vi "Pressure Generator.vi"() -> (2 "Trend Parameters":T1)   [LabVIEW 2015]
uses:
  Controls/Trend Parameters.ctl
panel:
  out "Frequency (Hz)":dbl[](array[numeric])
  out "DC":dbl[](array[numeric])
  out "Amplitude":dbl[](array[numeric])
  out "Noise Level":dbl[](array[numeric])
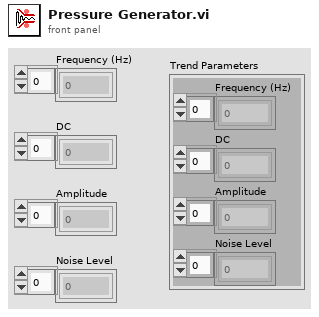
[diagram p1: front panel]
types:
  T1 = typedef "Trend Parameters.ctl" = cluster{"Frequency (Hz)":dbl[], "DC":dbl[], "Amplitude":dbl[], "Noise Level":dbl[]}
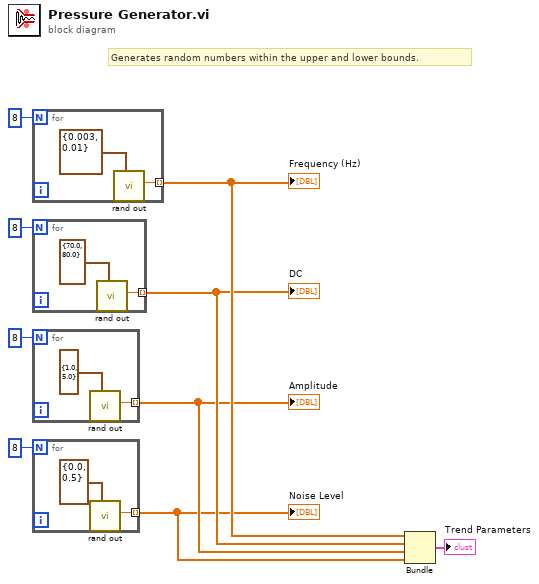
[diagram p0: block diagram]
diagram:
  # "Generates random numbers within the upper and lower bounds."
  n1 = for {
    N: 8 -> [_]
    tunnel: [w10] -> w5 mode=indexing
    n2 = call "rand out.vi"("Min/Max"=cluster{"Min":dbl, "Max":dbl} {"Min"=0.003, "Max"=0.01}) -> ("rand out"=w10:dbl)  [unwired: 10 in]
  }
  "Frequency (Hz)" <- w5
  n3 = for {
    N: 8 -> [_]
    tunnel: [w12] -> w4 mode=indexing
    n4 = call "rand out.vi"("Min/Max"=cluster{"Min":dbl, "Max":dbl} {"Min"=70.0, "Max"=80.0}) -> ("rand out"=w12:dbl)  [unwired: 10 in]
  }
  "DC" <- w4
  n5 = for {
    N: 8 -> [_]
    tunnel: [w14] -> w3 mode=indexing
    n6 = call "rand out.vi"("Min/Max"=cluster{"Min":dbl, "Max":dbl} {"Min"=1.0, "Max"=5.0}) -> ("rand out"=w14:dbl)  [unwired: 10 in]
  }
  "Amplitude" <- w3
  n7 = for {
    N: 8 -> [_]
    tunnel: [w16] -> w2 mode=indexing
    n8 = call "rand out.vi"("Min/Max"=cluster{"Min":dbl, "Max":dbl} {"Min"=0.0, "Max"=0.5}) -> ("rand out"=w16:dbl)  [unwired: 10 in]
  }
  "Noise Level" <- w2
  n9 = Bundle(w5, w4, w3, w2) -> (→"Trend Parameters":cluster{dbl[], dbl[], dbl[], dbl[]})  [unwired: 1 in]
